vi "波形图（两电压测量1）.vi"() -> ()   [LabVIEW 2017]
panel:
  out "波形图":cluster{i32, dbl, dbl[]}[](graph)
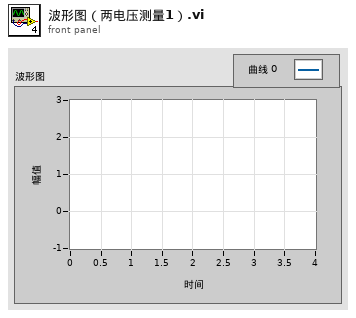
[diagram p1: front panel]
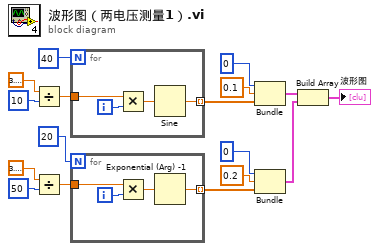
[diagram p0: block diagram]
diagram:
  n1 = Divide(x=3.141592653589793, y=10) -> (x/y=w14:dbl)
  n2 = Divide(x=3.141592653589793, y=50) -> (x/y=w6:dbl)
  n3 = for {
    N: 40 -> [_]
    tunnel: w14 -> [w21]
    tunnel: [w18] -> w11 mode=indexing
    i -> [w20]
    n4 = Multiply(x=w21, y=w20) -> (x*y=w19:dbl)
    n5 = Sine(x=w19) -> (sin(x)=w18:dbl)
  }
  n6 = for {
    N: 20 -> [_]
    tunnel: w6 -> [w25]
    tunnel: [w22] -> w3 mode=indexing
    i -> [w24]
    n7 = Multiply(x=w25, y=w24) -> (x*y=w23:dbl)
    n8 = Exponential (Arg) -1(1:w23) -> (0:w22:dbl)
  }
  n9 = Bundle(0, 0.1, w11) -> (w10:cluster{i32, dbl, dbl[]})  [unwired: 1 in]
  n10 = Bundle(0, 0.2, w3) -> (w2:cluster{i32, dbl, dbl[]})  [unwired: 1 in]
  n11 = Build Array(w10, w2) -> (→"波形图":cluster{i32, dbl, dbl[]}[])
